vi "Send Data SubVI.vi"(0 "Data Pin Task In":refnum<k21>, 1 "Sync Pin Task In":refnum<k21>, 2 "Write Pin Task In":refnum<k21>, 3 "Clear Pin Task In":refnum<k21>, 5 "Data":bool[](array[boolean])) -> (6 "Data Pin Task Out":refnum<k21>, 7 "Sync Pin Task Out":refnum<k21>, 8 "Write Pin Task Out":refnum<k21>, 9 "Clear Pin Task Out":refnum<k21>)   [LabVIEW 2020]
uses:
  <vilib>/DAQmx/write.llb/DAQmx Write (Digital Bool 1Line 1Point).vi
  <vilib>/DAQmx/miscellaneous.llb/DAQmx Fill In Error Info.vi
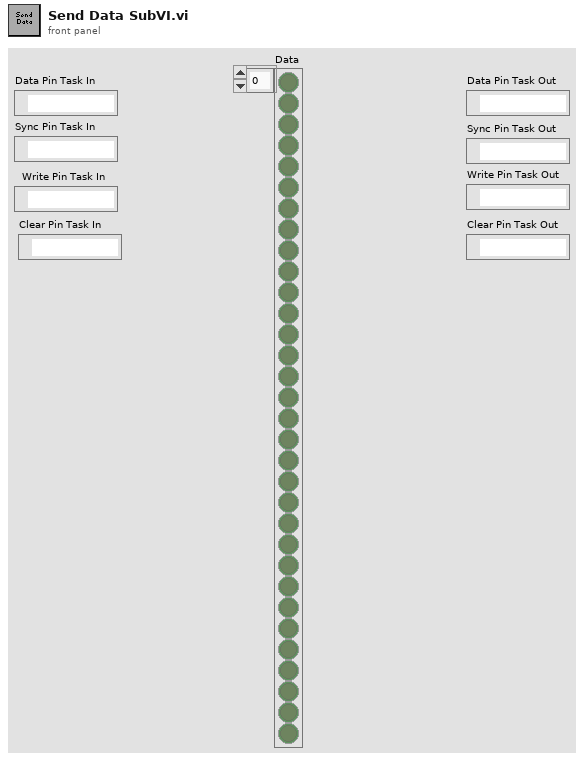
[diagram p1: front panel]
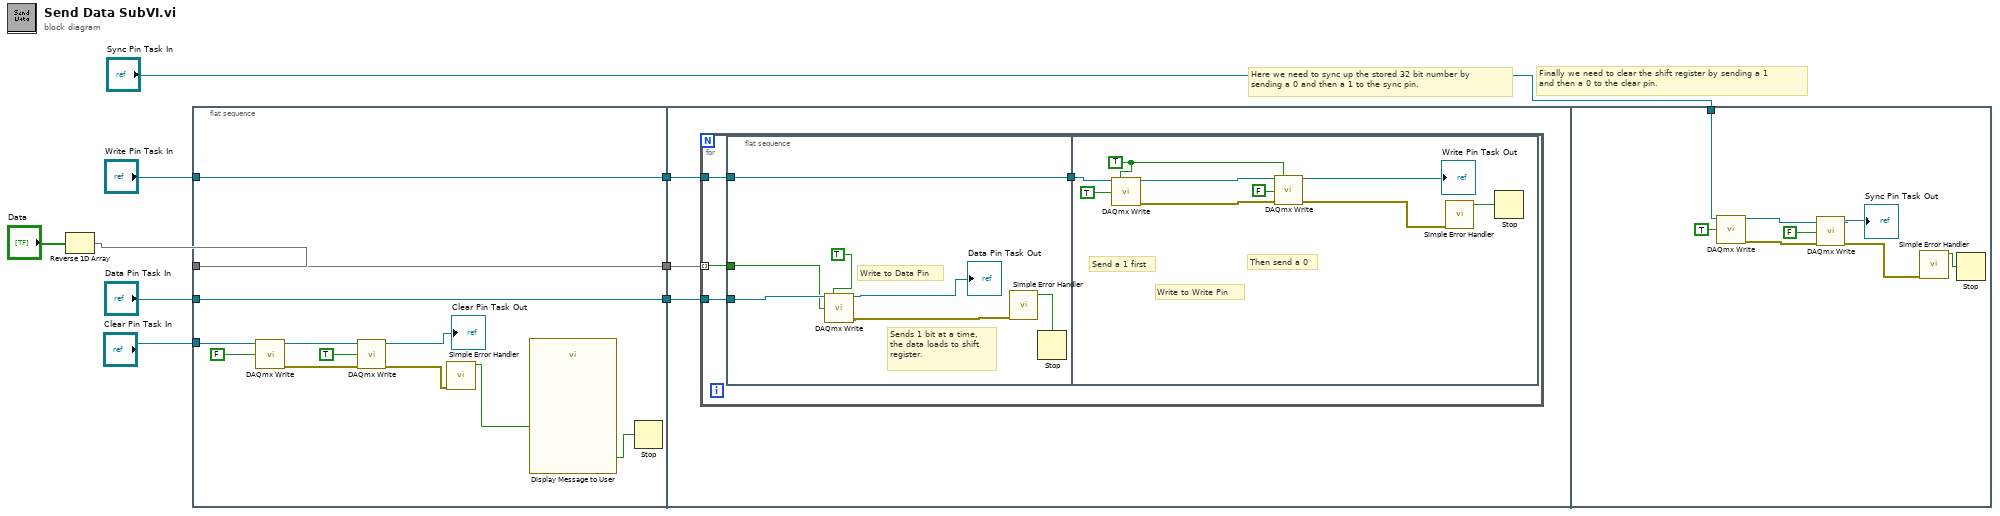
[diagram p0: block diagram]
diagram:
  # "Finally we need to clear the shift register by sending a 1\nand then a 0 to the clear pin."
  # "Here we need to sync up the stored 32 bit number by \nsending a 0 and then a 1 to the sync pin."
  n1 = Reverse 1D Array(array="Data") -> (reversed array=w2:bool[])
  n2 = flat-sequence {
    tunnel: w2 -> [w19]
    tunnel: "Data Pin Task In" -> [w20]
    tunnel: "Write Pin Task In" -> [w21]
    tunnel: [w21] -> w7
    tunnel: [w20] -> w6
    tunnel: [w19] -> w5
    tunnel: "Clear Pin Task In" -> [w12]
    tunnel: w7 -> [w24]
    tunnel: w6 -> [w23]
    tunnel: w5 -> [w22]
    tunnel: "Sync Pin Task In" -> [w46]
    frame #0 {
      n3 = call-poly <vilib>:"DAQmx Write.vi"("task/channels in"=w12, "data"=FALSE) -> ("task out"=w16:refnum<k21>, "error out"=w15:errorcluster)  [unwired: 11 in, 1 out]
      n4 = call-poly <vilib>:"DAQmx Write.vi"("task/channels in"=w16, "data"=TRUE, "error in"=w15) -> ("task out"=→"Clear Pin Task Out":refnum<k21>, "error out"=w13:errorcluster)  [unwired: 10 in, 1 out]
      n5 = call <vilib>:"Simple Error Handler.vi"("error in (no error)"=w13) -> ("error?"=w11:bool)  [unwired: 4 in, 4 out]
      n6 = call "Display Message to User"("Enable"=w11) -> ("OK"=w10:bool)  [unwired: 9 in, 1 out]
      n7 = Stop(stop? (T)=w10) -> ()
    }
    frame #1 {
      n8 = for {
        tunnel: w24 -> [w28]
        tunnel: w23 -> [w26]
        tunnel: w22 -> [w25] mode=indexing
        n9 = flat-sequence {
          tunnel: w28 -> [w35]
          tunnel: [w35] -> w27
          tunnel: w26 -> [w34]
          tunnel: w25 -> [w33]
          tunnel: w27 -> [w42]
          frame #0 {
            # "Sends 1 bit at a time,\nthe data loads to shift\nregister."
            # "Write to Data Pin"
            n10 = call-poly <vilib>:"DAQmx Write.vi"("task/channels in"=w34, "auto start"=TRUE, "data"=w33) -> ("task out"=→"Data Pin Task Out":refnum<k21>, "error out"=w30:errorcluster)  [unwired: 10 in, 1 out]
            n11 = call <vilib>:"Simple Error Handler.vi"("error in (no error)"=w30) -> ("error?"=w29:bool)  [unwired: 4 in, 4 out]
            n12 = Stop(stop? (T)=w29) -> ()
          }
          frame #1 {
            w37 = TRUE
            # "Then send a 0"
            # "Send a 1 first"
            # "Write to Write Pin"
            n13 = call-poly <vilib>:"DAQmx Write.vi"("task/channels in"=w42, "auto start"=w37, "data"=TRUE) -> ("task out"=w38:refnum<k21>, "error out"=w39:errorcluster)  [unwired: 10 in, 1 out]
            n14 = call-poly <vilib>:"DAQmx Write.vi"("task/channels in"=w38, "auto start"=w37, "data"=FALSE, "error in"=w39) -> ("task out"=→"Write Pin Task Out":refnum<k21>, "error out"=w40:errorcluster)  [unwired: 9 in, 1 out]
            n15 = call <vilib>:"Simple Error Handler.vi"("error in (no error)"=w40) -> ("error?"=w36:bool)  [unwired: 4 in, 4 out]
            n16 = Stop(stop? (T)=w36) -> ()
          }
        }
      }
    }
    frame #2 {
      n17 = call-poly <vilib>:"DAQmx Write.vi"("task/channels in"=w46, "data"=TRUE) -> ("task out"=w47:refnum<k21>, "error out"=w48:errorcluster)  [unwired: 11 in, 1 out]
      n18 = call-poly <vilib>:"DAQmx Write.vi"("task/channels in"=w47, "data"=FALSE, "error in"=w48) -> ("task out"=→"Sync Pin Task Out":refnum<k21>, "error out"=w49:errorcluster)  [unwired: 10 in, 1 out]
      n19 = call <vilib>:"Simple Error Handler.vi"("error in (no error)"=w49) -> ("error?"=w45:bool)  [unwired: 4 in, 4 out]
      n20 = Stop(stop? (T)=w45) -> ()
    }
  }
